vi "DWF MSO Query Analog Channel Characteristics.vi"(0 "Instrument Handle In":u32, 7 "Channel":string, 11 "Error In":errorcluster caption="Error In (no error)") -> (4 "Instrument Handle Out":u32, 6 "Input Impedance":i32(ring) items=["1 mega ohm", "50 ohms"], 8 "Bandwidth Limit":dbl, 15 "Error Out":errorcluster)   [LabVIEW 2015, in "DigilentWF.lvlib"]
doc: "Indicates the properties that control the electrical characteristics of the specified channel."
uses:
  <vilib>/DigilentWF/DigilentWF.lvlib
  dwf.dll
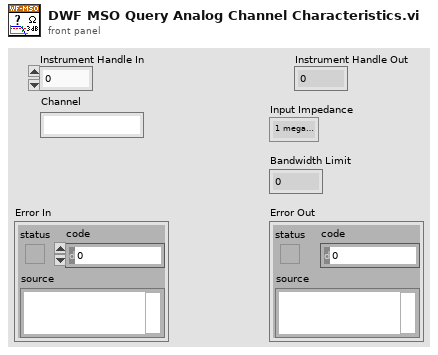
[diagram p1: front panel]
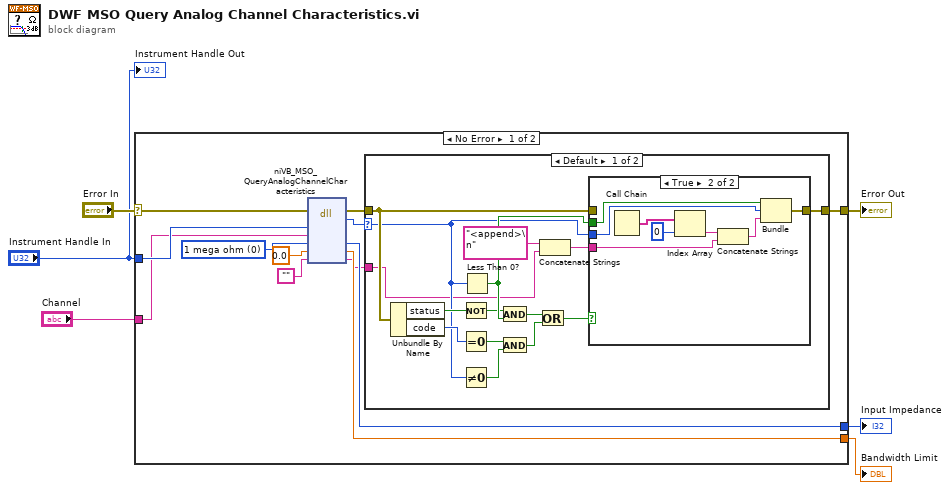
[diagram p0: block diagram]
diagram:
  n1 = case "outter_case" shown="No Error" "Error In" {
    selector: "Error In" -> [w18 w44]
    tunnel: [w15 w44] -> w5
    tunnel: "Instrument Handle In" -> [w14 _]
    tunnel: [w11 _] -> w3
    tunnel: [w10 _] -> w2
    tunnel: "Channel" -> [w7 _]
    frame No Error {
      w13 = 0 items=["1 mega ohm", "50 ohms"] ("Input Impedance")
      n2 = dll-call lib="dwf.*" fn="niVB_MSO_QueryAnalogChannelCharacteristics"(error in=w18, "InstrumentHandle"=w14, "Channel"=w7, "InputImpedance"=w13, "BandwidthLimit"=0.0 ("Bandwidth Limit"), "szError"="") -> (error out=w17:errorcluster, "return type"=w16:i32, "InputImpedance"=w11:i32, "BandwidthLimit"=w10:dbl, "szError"=w8:string)  [unwired: 4 in, 1 out]
      n3 = case "inner_case" shown="Default" w16 {
        selector: w16 -> [w23 _]
        tunnel: w17 -> [w24 w43]
        tunnel: [w20 w43] -> w15
        tunnel: w8 -> [w19 _]
        frame Default {
          n4 = Unbundle By Name(w24) -> ("status"=w28:bool, "code"=w32:i32)
          n5 = Not(x=w28) -> (.not. x?=w31:bool)
          n6 = Equal To 0?(x=w32) -> (x = 0?=w27:bool)
          n7 = Not Equal To 0?(x=w23) -> (x != 0?=w30:bool)
          n8 = Less Than 0?(x=w23) -> (x < 0?=w33:bool)
          n9 = And(x=w31, y=w33) -> (x .and. y?=w29:bool)
          n10 = And(x=w27, y=w30) -> (x .and. y?=w26:bool)
          n11 = Or(x=w29, y=w26) -> (x .or. y?=w25:bool)
          n12 = Concatenate Strings("<append>\n" ("string"), w19) -> (w22:string)
          n13 = case shown="True" w25 {
            tunnel: [w34 w41] -> w20
            tunnel: w23 -> [_ w40]
            tunnel: w33 -> [_ w39]
            tunnel: w24 -> [w34 _]
            tunnel: w22 -> [_ w35]
            frame False {
            }
            frame True {
              n14 = Call Chain() -> (call chain=w38:string[])
              n15 = Index Array(array=w38, index=0) -> (element=w37:string)
              n16 = Concatenate Strings(w37, w35) -> (w42:string)
              n17 = Bundle(w39, "return type"=w40, w42) -> (w41:cluster{bool, "return type":i32, string})  [unwired: 1 out]
            }
          }
        }
        frame 0 {
        }
      }
    }
    frame Error {
    }
  }
  "Error Out" <- w5
  "Input Impedance" <- w3
  "Bandwidth Limit" <- w2
  "Instrument Handle Out" <- "Instrument Handle In"
